vi "Enqueue.vi"(8 "error in":errorcluster, 11 "element":T1) -> (0 "error out":errorcluster)   [LabVIEW 2020]
uses:
  Controls/Queue.ctl
  Controls/Queue_Mode.ctl
  Controls/Queue_Action.ctl
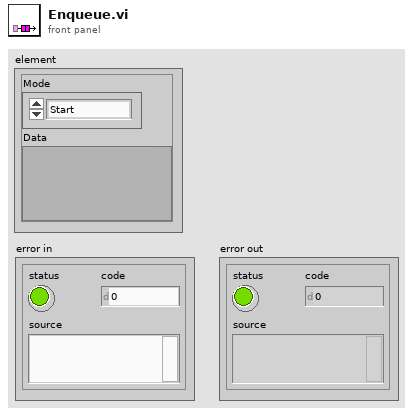
[diagram p1: front panel]
types:
  T1 = typedef "Queue.ctl" = cluster{"Mode":T2, "Data":variant}
  T2 = typedef "Queue_Mode.ctl" = enum16{"Start", "Stop"}
  T3 = typedef "Queue_Action.ctl" = enum16{"Get", "Set", "Release"}
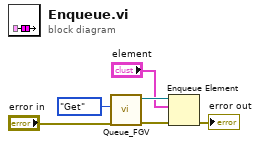
[diagram p0: block diagram]
diagram:
  n1 = call "Queue_FGV.vi"("error in"="error in", "Action"=Queue_Action."Get") -> ("error out"=w3:errorcluster, "Queue Out"=w5:refnum<queue>)  [unwired: 8 in]
  n2 = Enqueue Element(queue=w5, element="element", error in (no error)=w3) -> (error out=→"error out":errorcluster)  [unwired: 1 in, 2 out]
